vi "newImageEvent.vi"(8 "error in (no error)":errorcluster, 10 "Path":path, 11 "ImageStreamViewer in":refnum<class "ImageStreamViewer.lvclass">) -> (0 "error out":errorcluster, 3 "ImageStreamViewer out":refnum<class "ImageStreamViewer.lvclass">)   [LabVIEW 2009, in "Views.lvlib" / "Camera.lvlib" / "ImageStreamViewer.lvclass"]
uses:
  ImageStreamViewer.lvclass
  ImageStreamViewer.lvclass/ImageStreamViewer.ctl
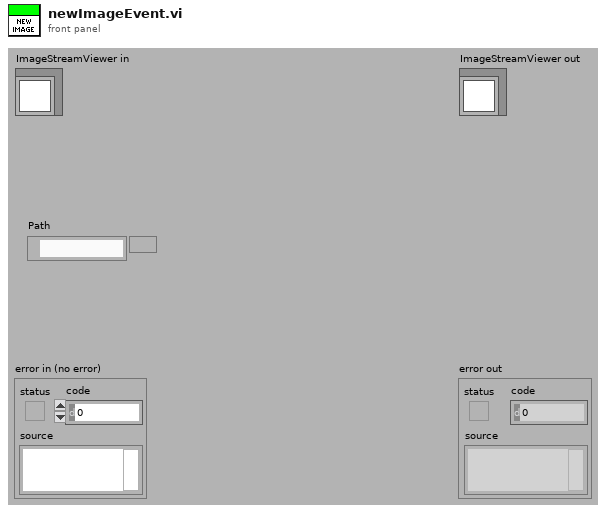
[diagram p1: front panel]
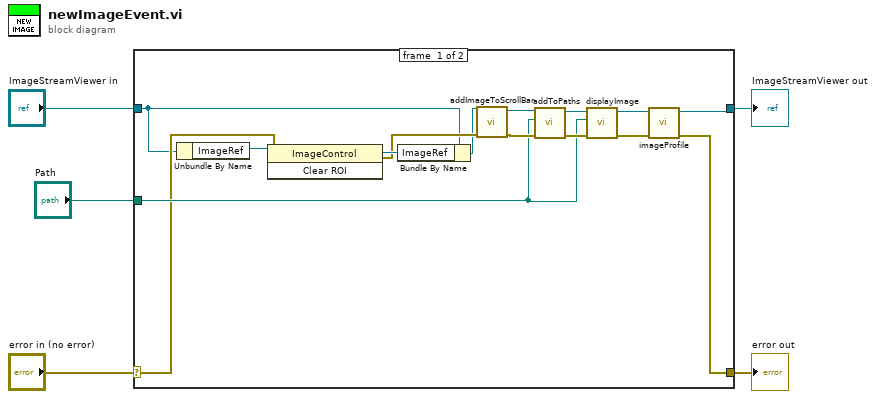
[diagram p0: block diagram]
diagram:
  n1 = case shown="No Error" "error in (no error)" {
    selector: "error in (no error)" -> [w9 w22]
    tunnel: [w13 w22] -> w4
    tunnel: [w12 w21] -> w2
    tunnel: "ImageStreamViewer in" -> [w7 w21]
    tunnel: "Path" -> [w16 _]
    frame #0 {
      n2 = Unbundle By Name(w7) -> ("ImageRef"=w11:refnum<vi>)
      n3 = invoke class="ImageControl" method="Clear ROI"(reference=w11, error in=w9) -> (reference out=w10:refnum<vi>, error out=w8:errorcluster)  [unwired: 1 in, 1 out]
      n4 = Bundle By Name(cluster=w7, "ImageRef"=w10) -> (w6:refnum<class "ImageStreamViewer.lvclass">)
      n5 = call "addImageToScrollBar.vi"("error in (no error)"=w8, "ImageStreamViewer in"=w6) -> ("error out"=w19:errorcluster, "ImageStreamViewer out"=w20:refnum<class "ImageStreamViewer.lvclass">)  [unwired: 8 in]
      n6 = call "addToPaths.vi"("error in (no error)"=w19, "Path"=w16, "ImageStreamViewer in"=w20) -> ("error out"=w17:errorcluster, "ImageStreamViewer out"=w18:refnum<class "ImageStreamViewer.lvclass">)  [unwired: 7 in]
      n7 = call "displayImage.vi"("error in (no error)"=w17, "Path"=w16, "ImageStreamViewer in"=w18) -> ("error out"=w14:errorcluster, "ImageStreamViewer out"=w15:refnum<class "ImageStreamViewer.lvclass">)  [unwired: 7 in]
      n8 = call "imageProfile.vi"("error in (no error)"=w14, "ImageStreamViewer in"=w15) -> ("error out"=w13:errorcluster, "ImageStreamViewer out"=w12:refnum<class "ImageStreamViewer.lvclass">)  [unwired: 8 in]
    }
    frame #1 {
    }
  }
  "error out" <- w4
  "ImageStreamViewer out" <- w2
